vi "compass.vi"() -> ()   [LabVIEW 2019, in "Nano33BLE-TiltCompensationSupport.lvlib"]
uses:
  types/compass_data.ctl
  types/xyz.ctl
  <vilib>/Instr/_visa.llb/VISA Configure Serial Port (Instr).vi
  Nano33BLE-TiltCompensationSupport.lvlib
panel:
  out "heading":dbl(graph)
  out "heading":dbl(knob)=10.401048171519527 scale=0.0..360.0
  in  "offset":dbl
  out "heading":dbl
  out "orientation":cluster{"X":dbl, "Y":dbl}[](graph)
  out "data out":T1
  in  "port":refnum<visa-resource-name>="COM3"
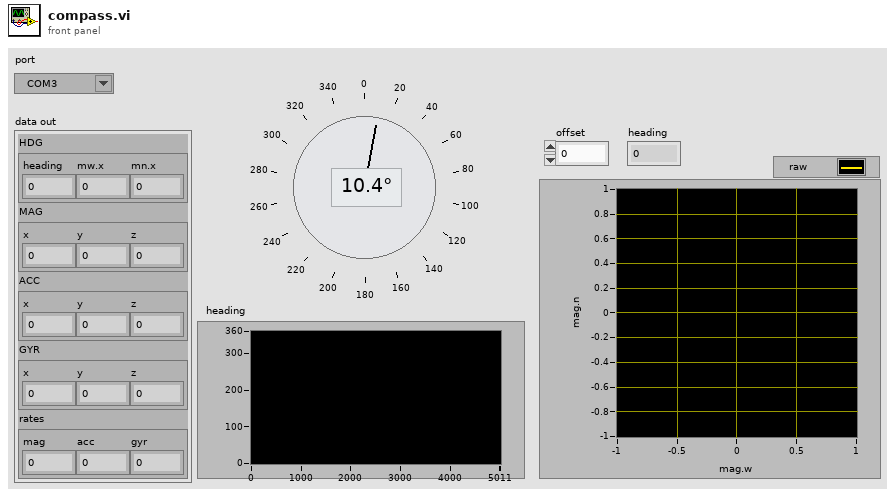
[diagram p1: front panel]
types:
  T1 = typedef "Nano33BLE-TiltCompensationSupport.lvlib/compass_data.ctl" = cluster{"HDG":cluster{"heading":dbl, "mw.x":dbl, "mn.x":dbl}, "MAG":T2, "ACC":T2, "GYR":T2, "rates":cluster{"mag":dbl, "acc":dbl, "gyr":dbl}}
  T2 = typedef "Nano33BLE-TiltCompensationSupport.lvlib/xyz.ctl" = cluster{"x":dbl, "y":dbl, "z":dbl}
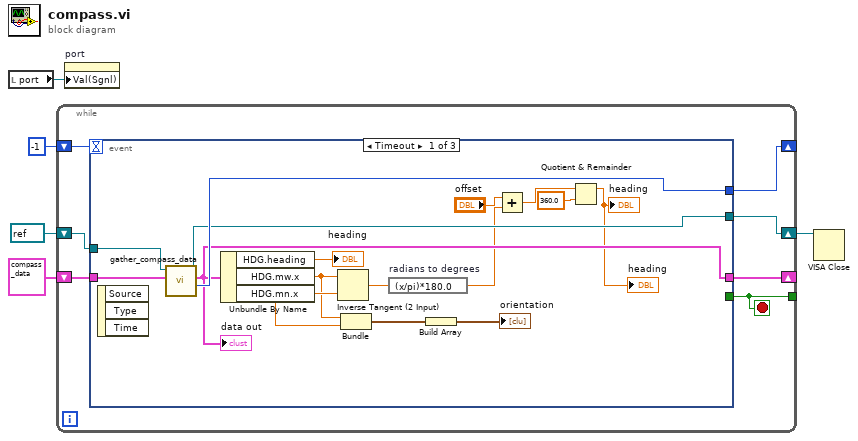
[diagram p0: block diagram]
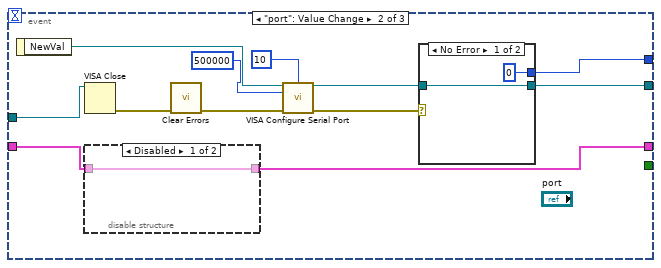
[diagram p2: hidden frame]
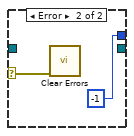
[diagram p4: hidden frame]
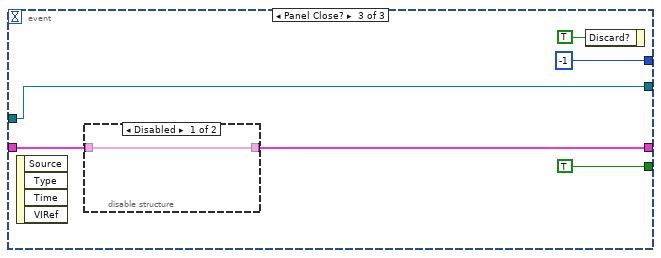
[diagram p5: hidden frame]
diagram:
  n1 = local read "port"() -> (w2:refnum<visa-resource-name>)
  n2 = while {
    tunnel: [w11] -> _
    shift-right: [w7] -> w3
    shift-left: refnum<visa-resource-name> refnum ("VISA resource name out") -> [w12]
    shift-right: [w8] -> _
    shift-left: -1 -> [w10]
    shift-right: [w6] -> _
    shift-left: T1 {"HDG"={"heading"=0.0, "mw.x"=0.0, "mn.x"=0.0}, "MAG"={"x"=0.0, "y"=0.0, "z"=0.0}, "ACC"={"x"=0.0, "y"=0.0, "z"=0.0}, "GYR"={"x"=0.0, "y"=0.0, "z"=0.0}, "rates"={"mag"=0.0, "acc"=0.0, "gyr"=0.0}} ("data out") -> [w9]
    stop <- w11 stop-if-true
    n3 = event shown="[0] Timeout" {
      selector: _ -> [_ _ _]
      dyn-events: _ -> [_ _ _]
      timeout: w10 -> [_ _ _]
      tunnel: w12 -> [w28 w38 w48]
      tunnel: [_ _ TRUE ("Discard?")] -> w11
      tunnel: w9 -> [w25 w29 w46]
      tunnel: [w27 w34 -1] -> w8
      tunnel: [w26 w33 w48] -> w7
      tunnel: [w24 w30 w47] -> w6
      event Timeout {
        n4 = event-data() -> ()  [unwired: 1 in, 3 out]
        n5 = call "gather_compass_data.vi"("data in"=w25, "VISA Refnum in"=w28) -> ("next timeout (ms)"=w27:i32, "data out"=w24:T1, "VISA Refnum out"=w26:refnum<visa-resource-name>)  [unwired: 7 in]
        "data out" <- w24
        n6 = Unbundle By Name(w24) -> ("HDG.heading"=→"heading":dbl, "HDG.mw.x"=w20:dbl, "HDG.mn.x"=w21:dbl)
        n7 = Inverse Tangent (2 Input)(1:w21, 2:w20) -> (0:w16:dbl)
        n8 = Bundle("mw.x"=w20, "mn.x"=w21) -> (w23:cluster{"mw.x":dbl, "mn.x":dbl})  [unwired: 1 in]
        n9 = expression code="(x/pi)*180.0" "radians to degrees"(w16) -> (w19:dbl)
        n10 = Build Array(w23) -> (→"orientation":cluster{"mw.x":dbl, "mn.x":dbl}[])
        n11 = Add(x="offset", y=w19) -> (x+y=w17:dbl)
        n12 = Quotient & Remainder(x=w17, y=360.0) -> (x-y*floor(x/y)=→"heading" →"heading":dbl)  [unwired: 1 out]
      }
      event "port": Value Change {
        n13 = event-data() -> ("NewVal"=w31:refnum<visa-resource-name>)  [unwired: 1 in]
        n14 = VISA Close(VISA resource name=w38) -> (error out=w37:errorcluster)  [unwired: 1 in]
        n15 = disable-structure shown="Disabled" {
          disable-tunnel: [w41 _] -> w30
          disable-tunnel: w29 -> [w41 _]
          frame Disabled {
          }
          frame Enabled {
          }
        }
        n16 = call <vilib>:"Clear Errors.vi"("error in (no error)"=w37) -> ("error out"=w36:errorcluster)  [unwired: 5 in, 1 out]
        n17 = call-poly "VISA Configure Serial Port"("VISA resource name"=w31, "termination char\n(0xA = '\\n' = LF)"=u8 10 ("termination char\n(0xA = '\\n' = LF)"), "baud rate (9600)"=u32 500000, "error in (no error)"=w36) -> ("VISA resource name out"=w32:refnum<visa-resource-name>, "error out"=w35:errorcluster)  [unwired: 10 in]
        n18 = case shown="No Error" w35 {
          selector: w35 -> [_ w45]
          tunnel: [0 -1] -> w34
          tunnel: [w42 _] -> w33
          tunnel: w32 -> [w42 _]
          frame No Error {
          }
          frame Error {
            n19 = call <vilib>:"Clear Errors.vi"("error in (no error)"=w45) -> ()  [unwired: 5 in, 2 out]
          }
        }
      }
      event Panel Close? {
        n20 = event-data() -> ()  [unwired: 1 in, 4 out]
        n21 = disable-structure shown="Disabled" {
          disable-tunnel: [w52 _] -> w47
          disable-tunnel: w46 -> [w52 _]
          frame Disabled {
          }
          frame Enabled {
          }
        }
        n22 = event-data("Discard?"=TRUE) -> ()  [unwired: 1 in, 1 out]
      }
    }
  }
  n23 = property on="port" class="VISAName"("Val(Sgnl)"=w2) -> ()  [unwired: 2 in, 2 out]
  n24 = VISA Close(VISA resource name=w3) -> ()  [unwired: 1 in, 1 out]
